vi "Obtain Request Events.vi"(8 "error in":errorcluster, 10 "Create New? (F)":bool) -> (0 "error out":errorcluster, 2 "RT Interpreter Manager Request Events":T1)   [LabVIEW 2021, in "RT Interpreter Manager.lvlib"]
doc: "This VI Obtains/Creates the Requests events that will be used for other modules to communicate with the module that owns this VI. These Requests events will be accessed only via Public API methods for this module.\n\n<b>NOTE</b>: The contents of this VI are automatically generated and modified by the <b>Tools > DQMH Consortium > DQMH</b> utilities. Consider using those utilities instead of making your own modifications to this VI.\n_____\nBased on DQMH Dev Tools: Project Template 7.1.2.1547."
uses:
  RT Interpreter Manager.lvlib
  Request Events--cluster.ctl
  Stop Argument--cluster.ctl
  Show Panel Argument--cluster.ctl
  Hide Panel Argument--cluster.ctl
  Get Module Execution Status Argument--cluster.ctl
  Show Diagram Argument--cluster.ctl
  Get Config Argument--cluster.ctl
  Open UDP Argument--cluster.ctl
  Start Read Messages from Host HL Argument--cluster.ctl
  New Host Connection Argument--cluster.ctl
  Send Message to Host Argument--cluster.ctl
  Libraries/UDP Comms/UDP Message--cluster.ctl
  Delete Host Connection Argument--cluster.ctl
  Libraries/UDP Comms/UDP Comms.lvlib
panel:
  # "NOTE: The contents of this VI are automatically generated and modified by the Tools > DQMH Consortium > DQMH utilities. Consider using those utilities instead of making your own modifications to this VI."
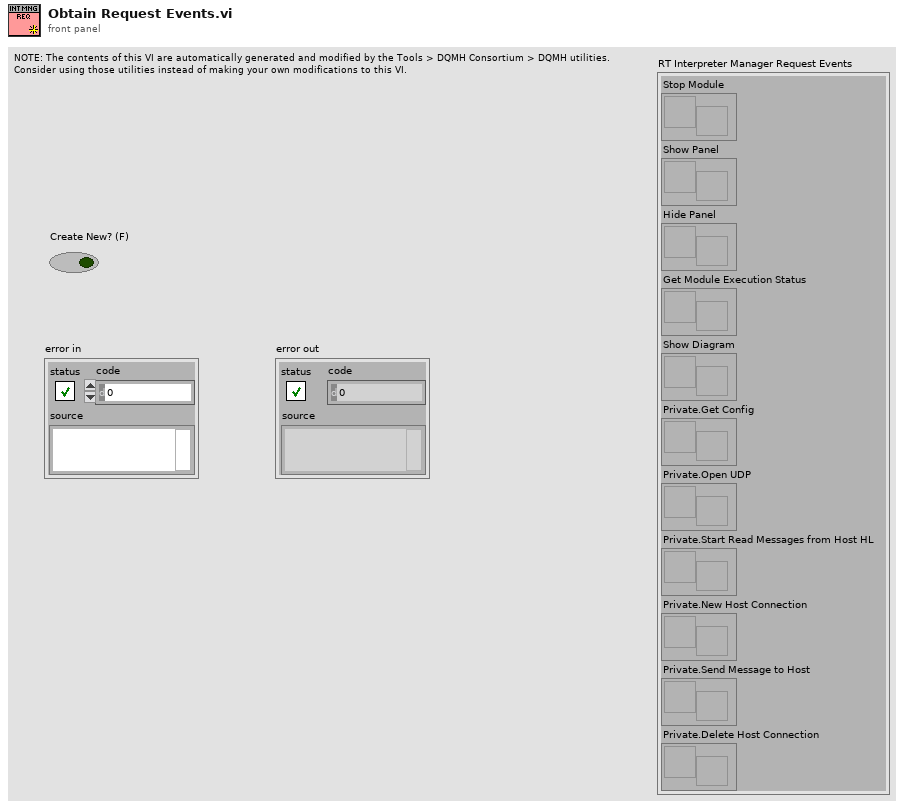
[diagram p1: front panel]
types:
  T1 = typedef "RT Interpreter Manager.lvlib/Request Events--cluster.ctl" = cluster{"Stop Module":refnum<user-event>, "Show Panel":refnum<user-event>, "Hide Panel":refnum<user-event>, "Get Module Execution Status":refnum<user-event>, "Show Diagram":refnum<user-event>, "Private.Get Config":refnum<user-event>, "Private.Open UDP":refnum<user-event>, "Private.Start Read Messages from Host HL":refnum<user-event>, "Private.New Host Connection":refnum<user-event>, "Private.Send Message to Host":refnum<user-event>, "Private.Delete Host Connection":refnum<user-event>}
  T2 = typedef "RT Interpreter Manager.lvlib/Send Message to Host Argument--cluster.ctl" = cluster{"UDP Message":T3, "Remote IP":string, "Remote UDP Listening Port":u16}
  T3 = typedef "UDP Comms.lvlib/UDP Message--cluster.ctl" = cluster{"Command":string, "Data":variant}
  T4 = typedef "RT Interpreter Manager.lvlib/New Host Connection Argument--cluster.ctl" = cluster{"Host Connection IP:Port:Master/Slave":string}
  T5 = typedef "RT Interpreter Manager.lvlib/Start Read Messages from Host HL Argument--cluster.ctl" = cluster{"Target UDP connection ID":refnum<k16>, "Polling Rate (ms)":i32}
  T6 = typedef "RT Interpreter Manager.lvlib/Open UDP Argument--cluster.ctl" = cluster{"Boolean":bool}
  T7 = typedef "RT Interpreter Manager.lvlib/Get Config Argument--cluster.ctl" = cluster{"Boolean":bool}
  T8 = typedef "RT Interpreter Manager.lvlib/Hide Panel Argument--cluster.ctl" = cluster{"Hide Panel?":bool}
  T9 = typedef "RT Interpreter Manager.lvlib/Show Panel Argument--cluster.ctl" = cluster{"Show Panel?":bool}
  T10 = typedef "RT Interpreter Manager.lvlib/Show Diagram Argument--cluster.ctl" = cluster{"Debug?":bool}
  T11 = typedef "RT Interpreter Manager.lvlib/Get Module Execution Status Argument--cluster.ctl" = cluster{"Running?":bool}
  T12 = typedef "RT Interpreter Manager.lvlib/Stop Argument--cluster.ctl" = cluster{"Origin":string, "Exit via Stop Module Req?":bool, "Wait for Module to stop?":bool}
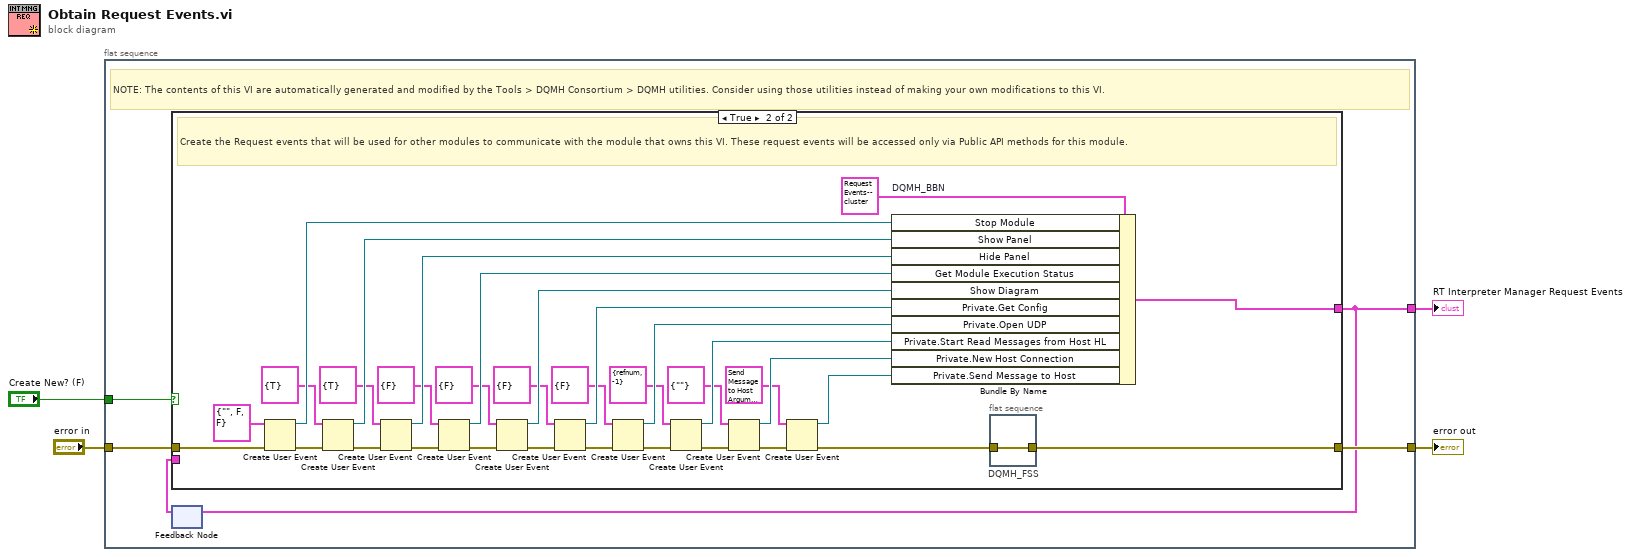
[diagram p0: block diagram]
diagram:
  n1 = flat-sequence {
    tunnel: [w9] -> w4
    tunnel: "error in" -> [w8]
    tunnel: [w6] -> w2
    tunnel: "Create New? (F)" -> [w5]
    frame #0 {
      # "NOTE: The contents of this VI are automatically generated and modified by the Tools > DQMH Consortium > DQMH utilities. Consider using those utilities instead of making your own modifications to this VI."
      n2 = feedback #1() -> (w7:T1)  [unwired: 1 in]
      n3 = case shown="True" w5 {
        tunnel: [w10 w35] -> w9
        tunnel: w8 -> [w10 w45]
        tunnel: [w11 w42] -> w6
        tunnel: w7 -> [w11 _]
        frame False {
          # "Obtain the Request events that were created in a previous call to this VI."
        }
        frame True {
          # "Create the Request events that will be used for other modules to communicate with the module that owns this VI. These request events will be accessed only via Public API methods for this module."
          n4 = Create User Event(user event datatype=T12 {"Origin"="", "Exit via Stop Module Req?"=FALSE, "Wait for Module to stop?"=FALSE} ("Stop Argument"), error in=w45) -> (user event=w43:refnum<user-event>, error out=w40:errorcluster)
          n5 = Create User Event(user event datatype=T9 {"Show Panel?"=TRUE} ("Show Panel Argument"), error in=w40) -> (user event=w39:refnum<user-event>, error out=w38:errorcluster)
          n6 = Create User Event(user event datatype=T8 {"Hide Panel?"=TRUE} ("Hide Panel Argument"), error in=w38) -> (user event=w37:refnum<user-event>, error out=w36:errorcluster)
          n7 = Create User Event(user event datatype=T11 {"Running?"=FALSE} ("Get Module Execution Status Argument"), error in=w36) -> (user event=w33:refnum<user-event>, error out=w34:errorcluster)
          n8 = Create User Event(user event datatype=T10 {"Debug?"=FALSE} ("Show Diagram Argument"), error in=w34) -> (user event=w30:refnum<user-event>, error out=w31:errorcluster)
          n9 = Create User Event(user event datatype=T7 {"Boolean"=FALSE} ("Get Config Argument"), error in=w31) -> (user event=w25:refnum<user-event>, error out=w26:errorcluster)
          n10 = Create User Event(user event datatype=T6 {"Boolean"=FALSE} ("Open UDP Argument"), error in=w26) -> (user event=w22:refnum<user-event>, error out=w23:errorcluster)
          n11 = Create User Event(user event datatype=T5 {"Target UDP connection ID"=refnum, "Polling Rate (ms)"=-1} ("Start Read Messages from Host HL Argument"), error in=w23) -> (user event=w19:refnum<user-event>, error out=w20:errorcluster)
          n12 = Create User Event(user event datatype=T4 {"Host Connection IP:Port:Master/Slave"=""} ("New Host Connection Argument"), error in=w20) -> (user event=w16:refnum<user-event>, error out=w17:errorcluster)
          n13 = Create User Event(user event datatype=T2 {"UDP Message"={"Command"="", "Data"=variant}, "Remote IP"="", "Remote UDP Listening Port"=0} ("Send Message to Host Argument"), error in=w17) -> (user event=w13:refnum<user-event>, error out=w14:errorcluster)
          n14 = Bundle By Name "DQMH_BBN"(cluster=T1 {"Stop Module"=refnum, "Show Panel"=refnum, "Hide Panel"=refnum, "Get Module Execution Status"=refnum, "Show Diagram"=refnum, "Private.Get Config"=refnum, "Private.Open UDP"=refnum, "Private.Start Read Messages from Host HL"=refnum, "Private.New Host Connection"=refnum, "Private.Send Message to Host"=refnum, "Private.Delete Host Connection"=refnum} ("output cluster"), "Stop Module"=w43, "Show Panel"=w39, "Hide Panel"=w37, "Get Module Execution Status"=w33, "Show Diagram"=w30, "Private.Get Config"=w25, "Private.Open UDP"=w22, "Private.Start Read Messages from Host HL"=w19, "Private.New Host Connection"=w16, "Private.Send Message to Host"=w13) -> (w42:T1)
          n15 = flat-sequence "DQMH_FSS" {
            tunnel: w14 -> [w46]
            tunnel: [w46] -> w35
            frame #0 {
            }
          }
        }
      }
      n16 = feedback-in #1(w6) -> ()
    }
  }
  "RT Interpreter Manager Request Events" <- w2
  "error out" <- w4
